vi "Calculate Velocity and Acceleration.vi"(10 "Loop Runtime (s)":dbl, 11 "Displacement (mm)":dbl) -> (2 "Acceleration (mm/s^2)":dbl, 3 "Velocity (mm/s)":dbl)   [LabVIEW 2017]
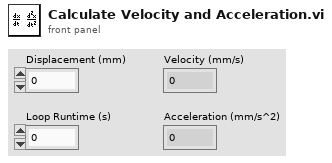
[diagram p1: front panel]
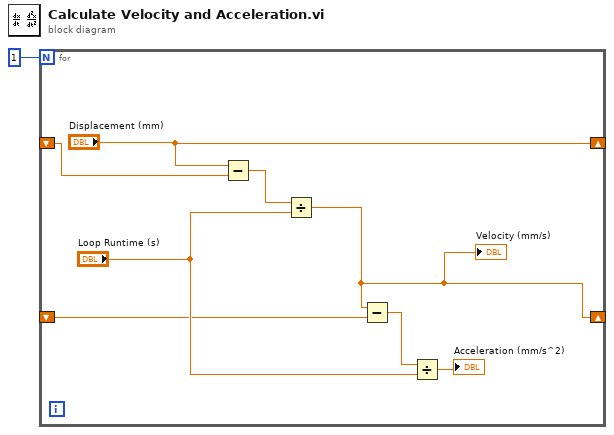
[diagram p0: block diagram]
diagram:
  n1 = for {
    N: 1 -> [_]
    shift-right: ["Displacement (mm)"] -> _
    shift-left: _ -> [w4]
    shift-right: [w2] -> _
    shift-left: _ -> [w3]
    n2 = Subtract(x="Displacement (mm)", y=w4) -> (x-y=w6:dbl)
    n3 = Divide(x=w6, y="Loop Runtime (s)") -> (x/y=w2:dbl)
    "Velocity (mm/s)" <- w2
    n4 = Subtract(x=w2, y=w3) -> (x-y=w7:dbl)
    n5 = Divide(x=w7, y="Loop Runtime (s)") -> (x/y=→"Acceleration (mm/s^2)":dbl)
  }
